vi "String To Number(U8).vi"(5 "String":string) -> (0 "Numeric(U8)":u8)   [LabVIEW 2017]
uses:
  <userlib>/_NEVSTOP/Communicable State Machine(CSM)/Communicable State Machine.lvlib
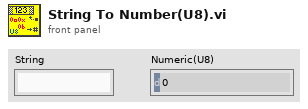
[diagram p1: front panel]
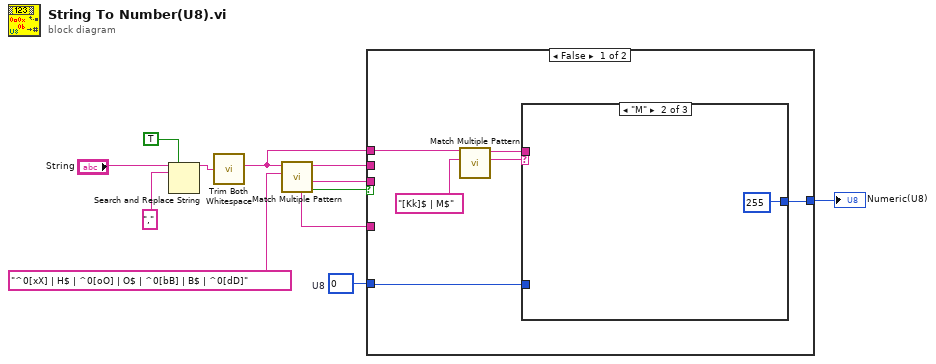
[diagram p0: block diagram]
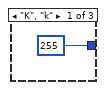
[diagram p2: hidden frame]
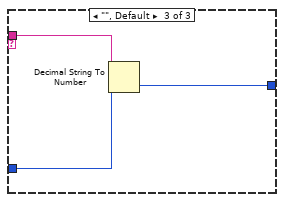
[diagram p3: hidden frame]
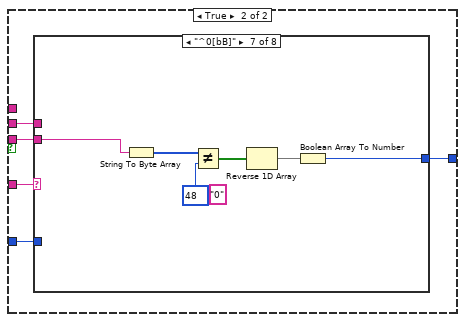
[diagram p4: hidden frame]
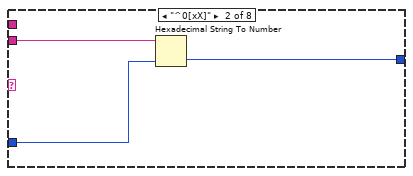
[diagram p6: hidden frame]
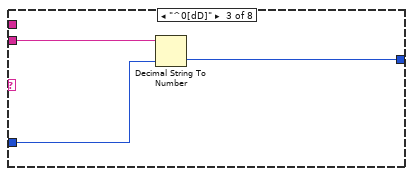
[diagram p7: hidden frame]
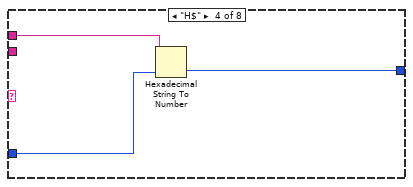
[diagram p8: hidden frame]
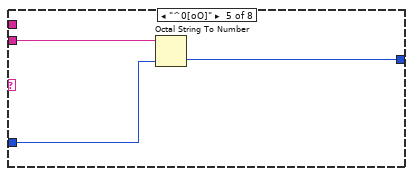
[diagram p9: hidden frame]
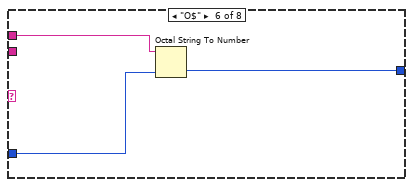
[diagram p10: hidden frame]
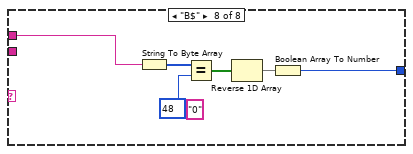
[diagram p11: hidden frame]
diagram:
  w1 = u8 0  # U8
  n1 = Search and Replace String(replace all?=TRUE ("replace all? (F)"), input string="String", search string=",") -> (result string=w9:string)  [unwired: 5 in, 3 out]
  n2 = call <userlib>:"Trim Both Whitespace.vi"("string"=w9) -> ("trimmed string"=w2:string)  [unwired: 1 in]
  n3 = call "Match Multiple Pattern.vi"("regular expression"="^0[xX] | H$ | ^0[oO] | O$ | ^0[bB] | B$ | ^0[dD]", "string"=w2) -> ("Found?"=w7:bool, "after substring"=w5:string, "before substring"=w4:string, "pattern matched"=w6:string)  [unwired: 5 in, 1 out]
  n4 = case shown="False" w7 {
    tunnel: w6 -> [_ w28]
    tunnel: w5 -> [_ w27]
    tunnel: w4 -> [_ w26]
    tunnel: [w13 w25] -> w3
    tunnel: w2 -> [w15 _]
    tunnel: w1 -> [w14 w24]
    frame False {
      n5 = call "Match Multiple Pattern.vi"("regular expression"="[Kk]$ | M$", "string"=w15) -> ("match substring"=w17:string, "before substring"=w16:string)  [unwired: 5 in, 3 out]
      n6 = case shown="\"M\"" w17 {
        tunnel: [u8 255 ("y") u8 255 ("y") w23] -> w13
        tunnel: w14 -> [_ _ w22]
        tunnel: w16 -> [_ _ w21]
        frame "K", "k" {
        }
        frame "M" {
        }
        frame "", Default {
          n7 = Decimal String To Number(string=w21, default (0L)=w22) -> (number=w23:u8)  [unwired: 1 in, 1 out]
        }
      }
    }
    frame True {
      n8 = case shown="\"^0[bB]\"" w28 {
        tunnel: w27 -> [_ w32 w35 _ w41 _ w49 _]
        tunnel: w26 -> [_ _ _ w37 _ w43 _ w53]
        tunnel: [w29 w31 w34 w38 w40 w44 w50 w56] -> w25
        tunnel: w24 -> [w29 w30 w33 w36 w39 w42 _ _]
        frame Default {
        }
        frame "^0[xX]" {
          n9 = Hexadecimal String To Number(string=w32, default (0uL)=w30) -> (number=w31:u8)  [unwired: 1 in, 1 out]
        }
        frame "^0[dD]" {
          n10 = Decimal String To Number(string=w35, default (0L)=w33) -> (number=w34:u8)  [unwired: 1 in, 1 out]
        }
        frame "H$" {
          n11 = Hexadecimal String To Number(string=w37, default (0uL)=w36) -> (number=w38:u8)  [unwired: 1 in, 1 out]
        }
        frame "^0[oO]" {
          n12 = Octal String To Number(2:w39, 4:w41) -> (0:w40:u8)  [unwired: 1 in, 1 out]
        }
        frame "O$" {
          n13 = Octal String To Number(2:w42, 4:w43) -> (0:w44:u8)  [unwired: 1 in, 1 out]
        }
        frame "^0[bB]" {
          (unwired) "0" ("search string")
          n14 = String To Byte Array(string=w49) -> (unsigned byte array=w48:u8[])
          n15 = Not Equal?(x=w48, y=u8 48) -> (x != y?=w46:bool[])
          n16 = Reverse 1D Array(array=w46) -> (reversed array=w45:bool[])
          n17 = Boolean Array To Number(Boolean array=w45) -> (number=w50:u8)
        }
        frame "B$" {
          (unwired) "0" ("search string")
          n18 = String To Byte Array(string=w53) -> (unsigned byte array=w55:u8[])
          n19 = Equal?(x=w55, y=u8 48) -> (x = y?=w54:bool[])
          n20 = Reverse 1D Array(array=w54) -> (reversed array=w52:bool[])
          n21 = Boolean Array To Number(Boolean array=w52) -> (number=w56:u8)
        }
      }
    }
  }
  "Numeric(U8)" <- w3
